vi "ReplaceInMatrix1.vi"(11 "Input Array":dbl[](array[numeric])) -> (0 "Output Array":dbl[][](array[numeric]))   [LabVIEW 2022 SP3]
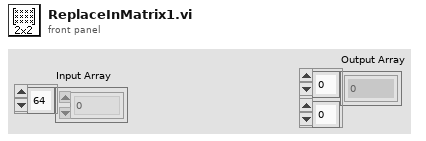
[diagram p1: front panel]
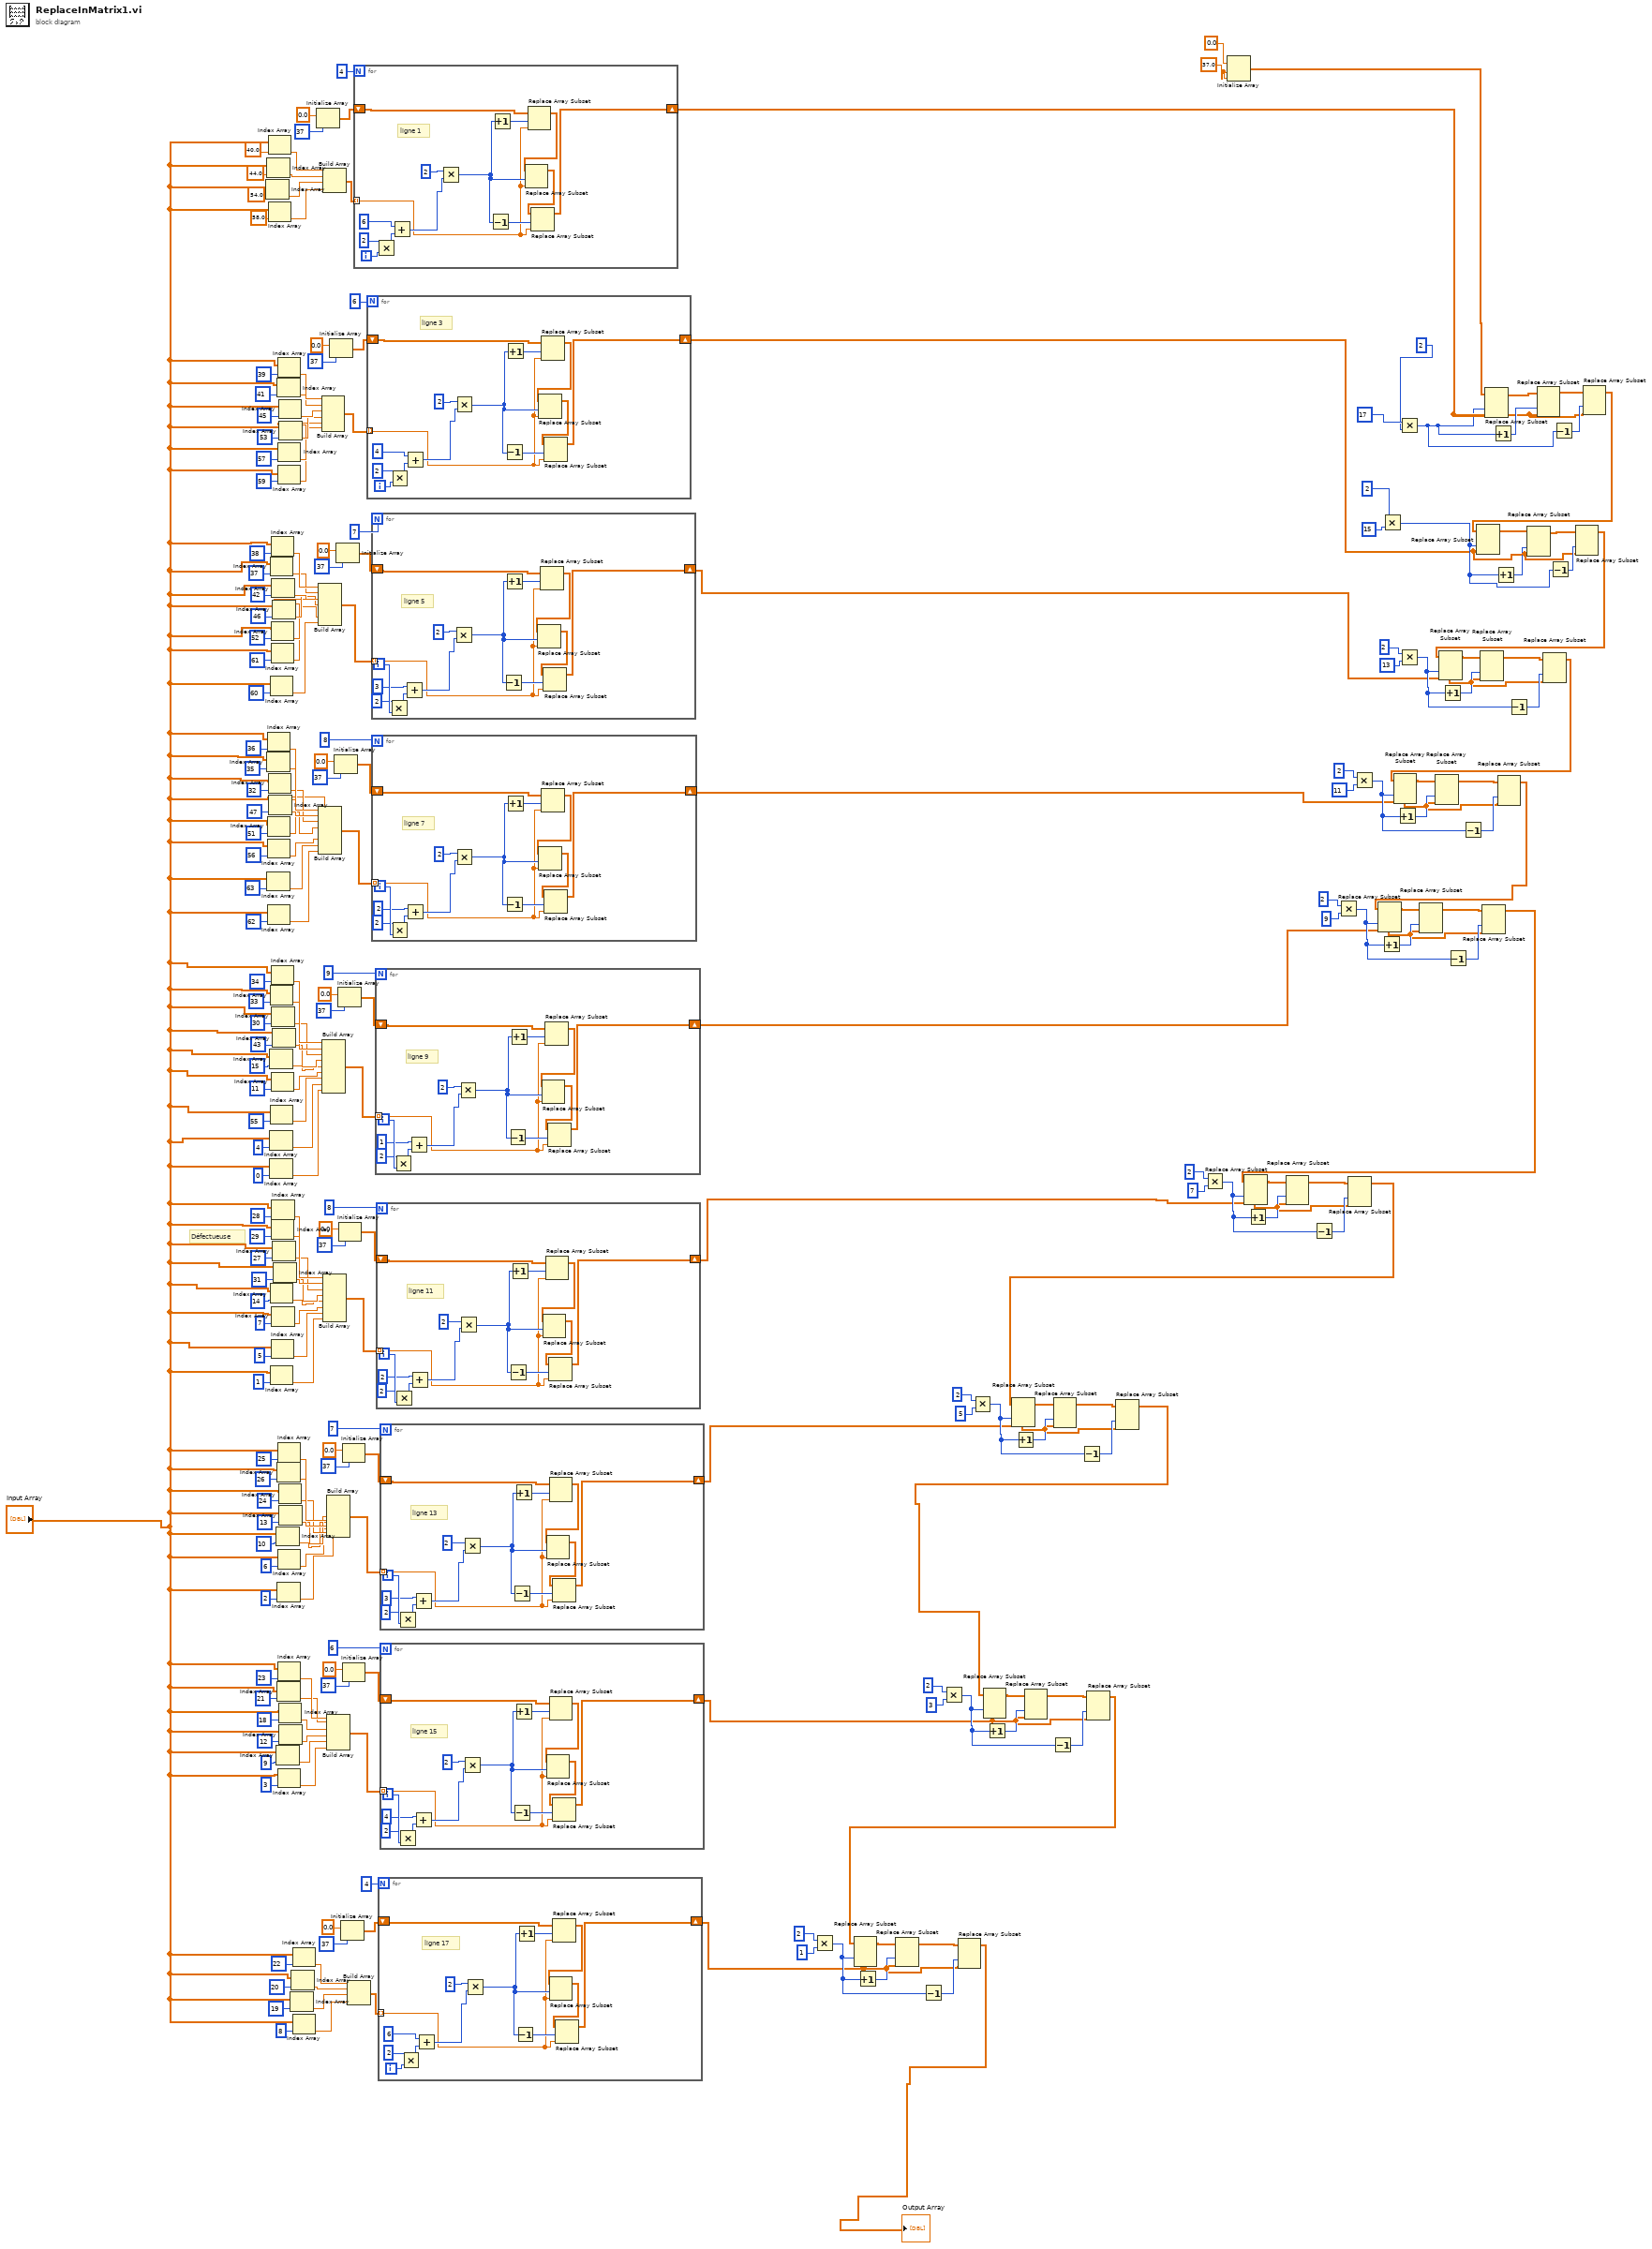
[diagram p0: block diagram]
diagram:
  w245 = 37.0
  # "Défectueuse"
  n1 = Index Array(array="Input Array", index=54.0 ("element")) -> (element=w226:dbl)
  n2 = Index Array(array="Input Array", index=44.0 ("element")) -> (element=w227:dbl)
  n3 = Index Array(array="Input Array", index=35) -> (element=w164:dbl)
  n4 = Index Array(array="Input Array", index=63) -> (element=w153:dbl)
  n5 = Index Array(array="Input Array", index=36) -> (element=w165:dbl)
  n6 = Index Array(array="Input Array", index=51) -> (element=w161:dbl)
  n7 = Index Array(array="Input Array", index=56) -> (element=w160:dbl)
  n8 = Index Array(array="Input Array", index=62) -> (element=w151:dbl)
  n9 = Index Array(array="Input Array", index=40.0 ("element")) -> (element=w228:dbl)
  n10 = Index Array(array="Input Array", index=58.0 ("element")) -> (element=w225:dbl)
  n11 = Index Array(array="Input Array", index=32) -> (element=w163:dbl)
  n12 = Index Array(array="Input Array", index=47) -> (element=w162:dbl)
  n13 = Index Array(array="Input Array", index=15) -> (element=w120:dbl)
  n14 = Index Array(array="Input Array", index=4) -> (element=w122:dbl)
  n15 = Index Array(array="Input Array", index=0) -> (element=w119:dbl)
  n16 = Index Array(array="Input Array", index=37) -> (element=w192:dbl)
  n17 = Index Array(array="Input Array", index=60) -> (element=w181:dbl)
  n18 = Index Array(array="Input Array", index=33) -> (element=w134:dbl)
  n19 = Index Array(array="Input Array", index=55) -> (element=w124:dbl)
  n20 = Index Array(array="Input Array", index=14) -> (element=w88:dbl)
  n21 = Index Array(array="Input Array", index=1) -> (element=w90:dbl)
  n22 = Index Array(array="Input Array", index=38) -> (element=w193:dbl)
  n23 = Index Array(array="Input Array", index=52) -> (element=w189:dbl)
  n24 = Index Array(array="Input Array", index=61) -> (element=w188:dbl)
  n25 = Index Array(array="Input Array", index=34) -> (element=w135:dbl)
  n26 = Index Array(array="Input Array", index=11) -> (element=w131:dbl)
  n27 = Index Array(array="Input Array", index=29) -> (element=w102:dbl)
  n28 = Index Array(array="Input Array", index=5) -> (element=w92:dbl)
  n29 = Index Array(array="Input Array", index=42) -> (element=w191:dbl)
  n30 = Index Array(array="Input Array", index=30) -> (element=w133:dbl)
  n31 = Index Array(array="Input Array", index=28) -> (element=w103:dbl)
  n32 = Index Array(array="Input Array", index=7) -> (element=w99:dbl)
  n33 = Index Array(array="Input Array", index=46) -> (element=w190:dbl)
  n34 = Index Array(array="Input Array", index=43) -> (element=w132:dbl)
  n35 = Index Array(array="Input Array", index=27) -> (element=w101:dbl)
  n36 = Index Array(array="Input Array", index=31) -> (element=w100:dbl)
  n37 = Index Array(array="Input Array", index=10) -> (element=w60:dbl)
  n38 = Index Array(array="Input Array", index=9) -> (element=w35:dbl)
  n39 = Index Array(array="Input Array", index=41) -> (element=w218:dbl)
  n40 = Index Array(array="Input Array", index=26) -> (element=w72:dbl)
  n41 = Index Array(array="Input Array", index=2) -> (element=w62:dbl)
  n42 = Index Array(array="Input Array", index=21) -> (element=w37:dbl)
  n43 = Index Array(array="Input Array", index=39) -> (element=w219:dbl)
  n44 = Index Array(array="Input Array", index=57) -> (element=w215:dbl)
  n45 = Index Array(array="Input Array", index=59) -> (element=w214:dbl)
  n46 = Index Array(array="Input Array", index=25) -> (element=w73:dbl)
  n47 = Index Array(array="Input Array", index=6) -> (element=w69:dbl)
  n48 = Index Array(array="Input Array", index=23) -> (element=w38:dbl)
  n49 = Index Array(array="Input Array", index=3) -> (element=w34:dbl)
  n50 = Index Array(array="Input Array", index=45) -> (element=w217:dbl)
  n51 = Index Array(array="Input Array", index=24) -> (element=w71:dbl)
  n52 = Index Array(array="Input Array", index=18) -> (element=w39:dbl)
  n53 = Index Array(array="Input Array", index=53) -> (element=w216:dbl)
  n54 = Index Array(array="Input Array", index=13) -> (element=w70:dbl)
  n55 = Index Array(array="Input Array", index=12) -> (element=w36:dbl)
  n56 = Index Array(array="Input Array", index=19) -> (element=w17:dbl)
  n57 = Index Array(array="Input Array", index=20) -> (element=w18:dbl)
  n58 = Index Array(array="Input Array", index=22) -> (element=w19:dbl)
  n59 = Index Array(array="Input Array", index=8) -> (element=w16:dbl)
  n60 = Initialize Array(0.0 ("element"), 37 ("dimension size")) -> (w236:dbl[])
  n61 = Build Array(w193, w192, w191, w190, w189, w188, w181) -> (w195:dbl[])
  n62 = Build Array(w165, w164, w163, w162, w161, w160, w153, w151) -> (w167:dbl[])
  n63 = Build Array(w219, w218, w217, w216, w215, w214) -> (w221:dbl[])
  n64 = Build Array(w135, w134, w133, w132, w120, w131, w124, w122, w119) -> (w137:dbl[])
  n65 = Build Array(w228, w227, w226, w225) -> (w235:dbl[])
  n66 = Build Array(w103, w102, w101, w100, w88, w99, w92, w90) -> (w105:dbl[])
  n67 = Build Array(w73, w72, w71, w70, w60, w69, w62) -> (w75:dbl[])
  n68 = Build Array(w38, w37, w39, w36, w35, w34) -> (w47:dbl[])
  n69 = Initialize Array(0.0 ("element"), 37 ("dimension size")) -> (w222:dbl[])
  n70 = Initialize Array(0.0 ("element"), 37 ("dimension size")) -> (w168:dbl[])
  n71 = Initialize Array(0.0 ("element"), 37 ("dimension size")) -> (w196:dbl[])
  n72 = Initialize Array(0.0 ("element"), 37 ("dimension size")) -> (w138:dbl[])
  n73 = Initialize Array(0.0 ("element"), 37 ("dimension size")) -> (w106:dbl[])
  n74 = Initialize Array(0.0 ("element"), 37 ("dimension size")) -> (w22:dbl[])
  n75 = Initialize Array(0.0 ("element"), 37 ("dimension size")) -> (w76:dbl[])
  n76 = Initialize Array(0.0 ("element"), 37 ("dimension size")) -> (w48:dbl[])
  n77 = Build Array(w19, w18, w17, w16) -> (w21:dbl[])
  n78 = for {
    N: 4 -> [_]
    tunnel: w235 -> [w249] mode=indexing
    shift-right: [w250] -> w233
    shift-left: w236 -> [w258]
    i -> [w257]
    # "ligne 1"
    n79 = Multiply(x=2, y=w257) -> (x*y=w255:i32)
    n80 = Add(x=6, y=w255) -> (x+y=w253:i32)
    n81 = Multiply(x=2, y=w253) -> (x*y=w252:i32)
    n82 = Decrement(x=w252) -> (x-1=w262:i32)
    n83 = Increment(x=w252) -> (x+1=w261:i32)
    n84 = Replace Array Subset(array=w258, new element=w249, index=w261) -> (w260:dbl[])
    n85 = Replace Array Subset(array=w260, new element=w249, index=w252) -> (w259:dbl[])
    n86 = Replace Array Subset(array=w259, new element=w249, index=w262) -> (w250:dbl[])
  }
  n87 = for {
    N: 6 -> [_]
    tunnel: w221 -> [w263] mode=indexing
    shift-right: [w264] -> w199
    shift-left: w222 -> [w272]
    i -> [w271]
    # "ligne 3"
    n88 = Multiply(x=2, y=w271) -> (x*y=w269:i32)
    n89 = Add(x=4, y=w269) -> (x+y=w267:i32)
    n90 = Multiply(x=2, y=w267) -> (x*y=w266:i32)
    n91 = Decrement(x=w266) -> (x-1=w276:i32)
    n92 = Increment(x=w266) -> (x+1=w275:i32)
    n93 = Replace Array Subset(array=w272, new element=w263, index=w275) -> (w274:dbl[])
    n94 = Replace Array Subset(array=w274, new element=w263, index=w266) -> (w273:dbl[])
    n95 = Replace Array Subset(array=w273, new element=w263, index=w276) -> (w264:dbl[])
  }
  n96 = for {
    N: 7 -> [_]
    tunnel: w195 -> [w277] mode=indexing
    shift-right: [w278] -> w171
    shift-left: w196 -> [w286]
    i -> [w285]
    # "ligne 5"
    n97 = Multiply(x=2, y=w285) -> (x*y=w283:i32)
    n98 = Add(x=3, y=w283) -> (x+y=w281:i32)
    n99 = Multiply(x=2, y=w281) -> (x*y=w280:i32)
    n100 = Decrement(x=w280) -> (x-1=w290:i32)
    n101 = Increment(x=w280) -> (x+1=w289:i32)
    n102 = Replace Array Subset(array=w286, new element=w277, index=w289) -> (w288:dbl[])
    n103 = Replace Array Subset(array=w288, new element=w277, index=w280) -> (w287:dbl[])
    n104 = Replace Array Subset(array=w287, new element=w277, index=w290) -> (w278:dbl[])
  }
  n105 = for {
    N: 8 -> [_]
    tunnel: w167 -> [w291] mode=indexing
    shift-right: [w292] -> w141
    shift-left: w168 -> [w300]
    i -> [w299]
    # "ligne 7"
    n106 = Multiply(x=2, y=w299) -> (x*y=w297:i32)
    n107 = Add(x=2, y=w297) -> (x+y=w295:i32)
    n108 = Multiply(x=2, y=w295) -> (x*y=w294:i32)
    n109 = Decrement(x=w294) -> (x-1=w304:i32)
    n110 = Increment(x=w294) -> (x+1=w303:i32)
    n111 = Replace Array Subset(array=w300, new element=w291, index=w303) -> (w302:dbl[])
    n112 = Replace Array Subset(array=w302, new element=w291, index=w294) -> (w301:dbl[])
    n113 = Replace Array Subset(array=w301, new element=w291, index=w304) -> (w292:dbl[])
  }
  n114 = for {
    N: 9 -> [_]
    tunnel: w137 -> [w305] mode=indexing
    shift-right: [w306] -> w109
    shift-left: w138 -> [w314]
    i -> [w313]
    # "ligne 9"
    n115 = Multiply(x=2, y=w313) -> (x*y=w311:i32)
    n116 = Add(x=1, y=w311) -> (x+y=w309:i32)
    n117 = Multiply(x=2, y=w309) -> (x*y=w308:i32)
    n118 = Decrement(x=w308) -> (x-1=w318:i32)
    n119 = Increment(x=w308) -> (x+1=w317:i32)
    n120 = Replace Array Subset(array=w314, new element=w305, index=w317) -> (w316:dbl[])
    n121 = Replace Array Subset(array=w316, new element=w305, index=w308) -> (w315:dbl[])
    n122 = Replace Array Subset(array=w315, new element=w305, index=w318) -> (w306:dbl[])
  }
  n123 = for {
    N: 8 -> [_]
    tunnel: w105 -> [w319] mode=indexing
    shift-right: [w320] -> w79
    shift-left: w106 -> [w328]
    i -> [w327]
    # "ligne 11"
    n124 = Multiply(x=2, y=w327) -> (x*y=w325:i32)
    n125 = Add(x=2, y=w325) -> (x+y=w323:i32)
    n126 = Multiply(x=2, y=w323) -> (x*y=w322:i32)
    n127 = Decrement(x=w322) -> (x-1=w332:i32)
    n128 = Increment(x=w322) -> (x+1=w331:i32)
    n129 = Replace Array Subset(array=w328, new element=w319, index=w331) -> (w330:dbl[])
    n130 = Replace Array Subset(array=w330, new element=w319, index=w322) -> (w329:dbl[])
    n131 = Replace Array Subset(array=w329, new element=w319, index=w332) -> (w320:dbl[])
  }
  n132 = for {
    N: 4 -> [_]
    tunnel: w21 -> [w333] mode=indexing
    shift-right: [w334] -> w2
    shift-left: w22 -> [w342]
    i -> [w341]
    # "ligne 17"
    n133 = Multiply(x=2, y=w341) -> (x*y=w339:i32)
    n134 = Add(x=6, y=w339) -> (x+y=w337:i32)
    n135 = Multiply(x=2, y=w337) -> (x*y=w336:i32)
    n136 = Decrement(x=w336) -> (x-1=w346:i32)
    n137 = Increment(x=w336) -> (x+1=w345:i32)
    n138 = Replace Array Subset(array=w342, new element=w333, index=w345) -> (w344:dbl[])
    n139 = Replace Array Subset(array=w344, new element=w333, index=w336) -> (w343:dbl[])
    n140 = Replace Array Subset(array=w343, new element=w333, index=w346) -> (w334:dbl[])
  }
  n141 = for {
    N: 7 -> [_]
    tunnel: w75 -> [w347] mode=indexing
    shift-right: [w348] -> w52
    shift-left: w76 -> [w356]
    i -> [w355]
    # "ligne 13"
    n142 = Multiply(x=2, y=w355) -> (x*y=w353:i32)
    n143 = Add(x=3, y=w353) -> (x+y=w351:i32)
    n144 = Multiply(x=2, y=w351) -> (x*y=w350:i32)
    n145 = Decrement(x=w350) -> (x-1=w360:i32)
    n146 = Increment(x=w350) -> (x+1=w359:i32)
    n147 = Replace Array Subset(array=w356, new element=w347, index=w359) -> (w358:dbl[])
    n148 = Replace Array Subset(array=w358, new element=w347, index=w350) -> (w357:dbl[])
    n149 = Replace Array Subset(array=w357, new element=w347, index=w360) -> (w348:dbl[])
  }
  n150 = for {
    N: 6 -> [_]
    tunnel: w47 -> [w361] mode=indexing
    shift-right: [w362] -> w25
    shift-left: w48 -> [w370]
    i -> [w369]
    # "ligne 15"
    n151 = Multiply(x=2, y=w369) -> (x*y=w367:i32)
    n152 = Add(x=4, y=w367) -> (x+y=w365:i32)
    n153 = Multiply(x=2, y=w365) -> (x*y=w364:i32)
    n154 = Decrement(x=w364) -> (x-1=w374:i32)
    n155 = Increment(x=w364) -> (x+1=w373:i32)
    n156 = Replace Array Subset(array=w370, new element=w361, index=w373) -> (w372:dbl[])
    n157 = Replace Array Subset(array=w372, new element=w361, index=w364) -> (w371:dbl[])
    n158 = Replace Array Subset(array=w371, new element=w361, index=w374) -> (w362:dbl[])
  }
  n159 = Multiply(x=2, y=1 ("index (row)")) -> (x*y=w5:i32)
  n160 = Increment(x=w5) -> (x+1=w4:i32)
  n161 = Decrement(x=w5) -> (x-1=w6:i32)
  n162 = Multiply(x=2, y=3 ("index (row)")) -> (x*y=w28:i32)
  n163 = Multiply(x=2, y=5 ("index (row)")) -> (x*y=w54:i32)
  n164 = Increment(x=w28) -> (x+1=w27:i32)
  n165 = Increment(x=w54) -> (x+1=w53:i32)
  n166 = Decrement(x=w28) -> (x-1=w29:i32)
  n167 = Decrement(x=w54) -> (x-1=w55:i32)
  n168 = Multiply(x=2, y=7 ("index (row)")) -> (x*y=w82:i32)
  n169 = Initialize Array(0.0, w245, w245) -> (w244:dbl[][])
  n170 = Increment(x=w82) -> (x+1=w81:i32)
  n171 = Decrement(x=w82) -> (x-1=w83:i32)
  n172 = Multiply(x=2, y=9 ("index (row)")) -> (x*y=w112:i32)
  n173 = Multiply(x=2, y=11 ("index (row)")) -> (x*y=w144:i32)
  n174 = Increment(x=w112) -> (x+1=w111:i32)
  n175 = Multiply(x=2, y=15 ("index (row)")) -> (x*y=w201:i32)
  n176 = Increment(x=w144) -> (x+1=w143:i32)
  n177 = Multiply(x=17 ("index (row)"), y=2 ("index (row)")) -> (x*y=w206:i32)
  n178 = Multiply(x=2, y=13 ("index (row)")) -> (x*y=w173:i32)
  n179 = Increment(x=w173) -> (x+1=w172:i32)
  n180 = Decrement(x=w112) -> (x-1=w113:i32)
  n181 = Decrement(x=w144) -> (x-1=w145:i32)
  n182 = Replace Array Subset(array=w244, new element=w233, index (col)=w206) -> (w243:dbl[][])  [unwired: 1 in]
  n183 = Increment(x=w206) -> (x+1=w242:i32)
  n184 = Increment(x=w201) -> (x+1=w202:i32)
  n185 = Decrement(x=w173) -> (x-1=w174:i32)
  n186 = Replace Array Subset(array=w243, new element=w233, index (col)=w242) -> (w241:dbl[][])  [unwired: 1 in]
  n187 = Decrement(x=w201) -> (x-1=w200:i32)
  n188 = Decrement(x=w206) -> (x-1=w240:i32)
  n189 = Replace Array Subset(array=w241, new element=w233, index (col)=w240) -> (w239:dbl[][])  [unwired: 1 in]
  n190 = Replace Array Subset(array=w239, new element=w199, index (col)=w201) -> (w204:dbl[][])  [unwired: 1 in]
  n191 = Replace Array Subset(array=w204, new element=w199, index (col)=w202) -> (w203:dbl[][])  [unwired: 1 in]
  n192 = Replace Array Subset(array=w203, new element=w199, index (col)=w200) -> (w177:dbl[][])  [unwired: 1 in]
  n193 = Replace Array Subset(array=w177, new element=w171, index (col)=w173) -> (w176:dbl[][])  [unwired: 1 in]
  n194 = Replace Array Subset(array=w176, new element=w171, index (col)=w172) -> (w175:dbl[][])  [unwired: 1 in]
  n195 = Replace Array Subset(array=w175, new element=w171, index (col)=w174) -> (w142:dbl[][])  [unwired: 1 in]
  n196 = Replace Array Subset(array=w142, new element=w141, index (col)=w144) -> (w147:dbl[][])  [unwired: 1 in]
  n197 = Replace Array Subset(array=w147, new element=w141, index (col)=w143) -> (w146:dbl[][])  [unwired: 1 in]
  n198 = Replace Array Subset(array=w146, new element=w141, index (col)=w145) -> (w110:dbl[][])  [unwired: 1 in]
  n199 = Replace Array Subset(array=w110, new element=w109, index (col)=w112) -> (w115:dbl[][])  [unwired: 1 in]
  n200 = Replace Array Subset(array=w115, new element=w109, index (col)=w111) -> (w114:dbl[][])  [unwired: 1 in]
  n201 = Replace Array Subset(array=w114, new element=w109, index (col)=w113) -> (w80:dbl[][])  [unwired: 1 in]
  n202 = Replace Array Subset(array=w80, new element=w79, index (col)=w82) -> (w85:dbl[][])  [unwired: 1 in]
  n203 = Replace Array Subset(array=w85, new element=w79, index (col)=w81) -> (w84:dbl[][])  [unwired: 1 in]
  n204 = Replace Array Subset(array=w84, new element=w79, index (col)=w83) -> (w51:dbl[][])  [unwired: 1 in]
  n205 = Replace Array Subset(array=w51, new element=w52, index (col)=w54) -> (w57:dbl[][])  [unwired: 1 in]
  n206 = Replace Array Subset(array=w57, new element=w52, index (col)=w53) -> (w56:dbl[][])  [unwired: 1 in]
  n207 = Replace Array Subset(array=w56, new element=w52, index (col)=w55) -> (w26:dbl[][])  [unwired: 1 in]
  n208 = Replace Array Subset(array=w26, new element=w25, index (col)=w28) -> (w31:dbl[][])  [unwired: 1 in]
  n209 = Replace Array Subset(array=w31, new element=w25, index (col)=w27) -> (w30:dbl[][])  [unwired: 1 in]
  n210 = Replace Array Subset(array=w30, new element=w25, index (col)=w29) -> (w3:dbl[][])  [unwired: 1 in]
  n211 = Replace Array Subset(array=w3, new element=w2, index (col)=w5) -> (w8:dbl[][])  [unwired: 1 in]
  n212 = Replace Array Subset(array=w8, new element=w2, index (col)=w4) -> (w7:dbl[][])  [unwired: 1 in]
  n213 = Replace Array Subset(array=w7, new element=w2, index (col)=w6) -> (→"Output Array":dbl[][])  [unwired: 1 in]
